vi "fftw__malloc_poly.vi"   [LabVIEW 2020, in "FFTWDLL.lvlib"]
doc: "Allocate FFTW aligned memory block."
uses:
  FFTWDLL.lvlib
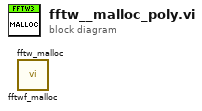
[diagram p0: block diagram]
diagram:
  n1 = call "fftwf_malloc.vi"() -> ()  [unwired: 10 in, 2 out]
  n2 = call "fftw_malloc.vi"() -> ()  [unwired: 10 in, 2 out]
